vi "Teleop.vi"(10 "Match Info":T7={"Autonomous Elapsed Seconds"=0.0, "TeleOp Elapsed Seconds"=0.0, "Disabled Elapsed Seconds"=0.0, "Visited Autonomous"=FALSE, "Visited TeleOp"=FALSE, "Visited Disabled"=FALSE, "Autonomous Settings"={"Autonomous Style"=enum."Independent", "VI Refnum"=refnum}}, 11 "Call Context":T8) -> ()   [LabVIEW 2015]
doc: "This VI is called for each TeleOp packet received from the DS where the robot is not disabled. It is often used to read from the joysticks and update I/O or to update setpoints for timed control loops. It should complete and return within 20 milliseconds or it may miss DS packets."
uses:
  <vilib>/Rock Robotics/WPI/DriverStation/WPI_DriverStationDerivedRobotMode.ctl
  <vilib>/Rock Robotics/WPI/DriverStation/WPI_DriverStationMatch Info.ctl
  <vilib>/Rock Robotics/Network Tables/NT Read Boolean.vi
  <vilib>/Rock Robotics/Network Tables/NT Read Number.vi
  <vilib>/Rock Robotics/WPI/Utilities/WPI_GetSetVariantRefNum.vi
  <vilib>/Rock Robotics/Network Tables/NT Write Boolean Array.vi
  <vilib>/Rock Robotics/Network Tables/NT Write Numeric Array.vi
  <vilib>/functionblocks/Counter/Timer On Delay/Timer On Delay.vi
  <vilib>/functionblocks/Counter/Pulse Timer/Pulse Timer.vi
  Robot Global Data.vi
  Global 1.vi
  Global 2.vi
  <vilib>/Rock Robotics/Network Tables/NT Write Boolean.vi
  <vilib>/functionblocks/FB Core/FB Core.xnode
  <vilib>/functionblocks/NI_FunctionBlock Libraries.lvlib
panel:
  out "Catapult":T1
  out "DriveTrain Analog":T2
  out "Camera and Joystick Flip Control":T3
  out "Joystick 0 Buttons":T4
  out "Joystick 1 Buttons":T5
  out "Pneumatic Block #1":T6
  out "Arm Angle Ref":dbl
  out "Arm Difference (PID Input)":dbl
  out "Arm Angle":dbl
  out "Sample Slider 0":dbl(slide) scale=0.0..5.0
  out "Sample Boolean 1":bool
  out "Sample Boolean 0":bool
  # "Fwd/Rev"
  # "Left Right"
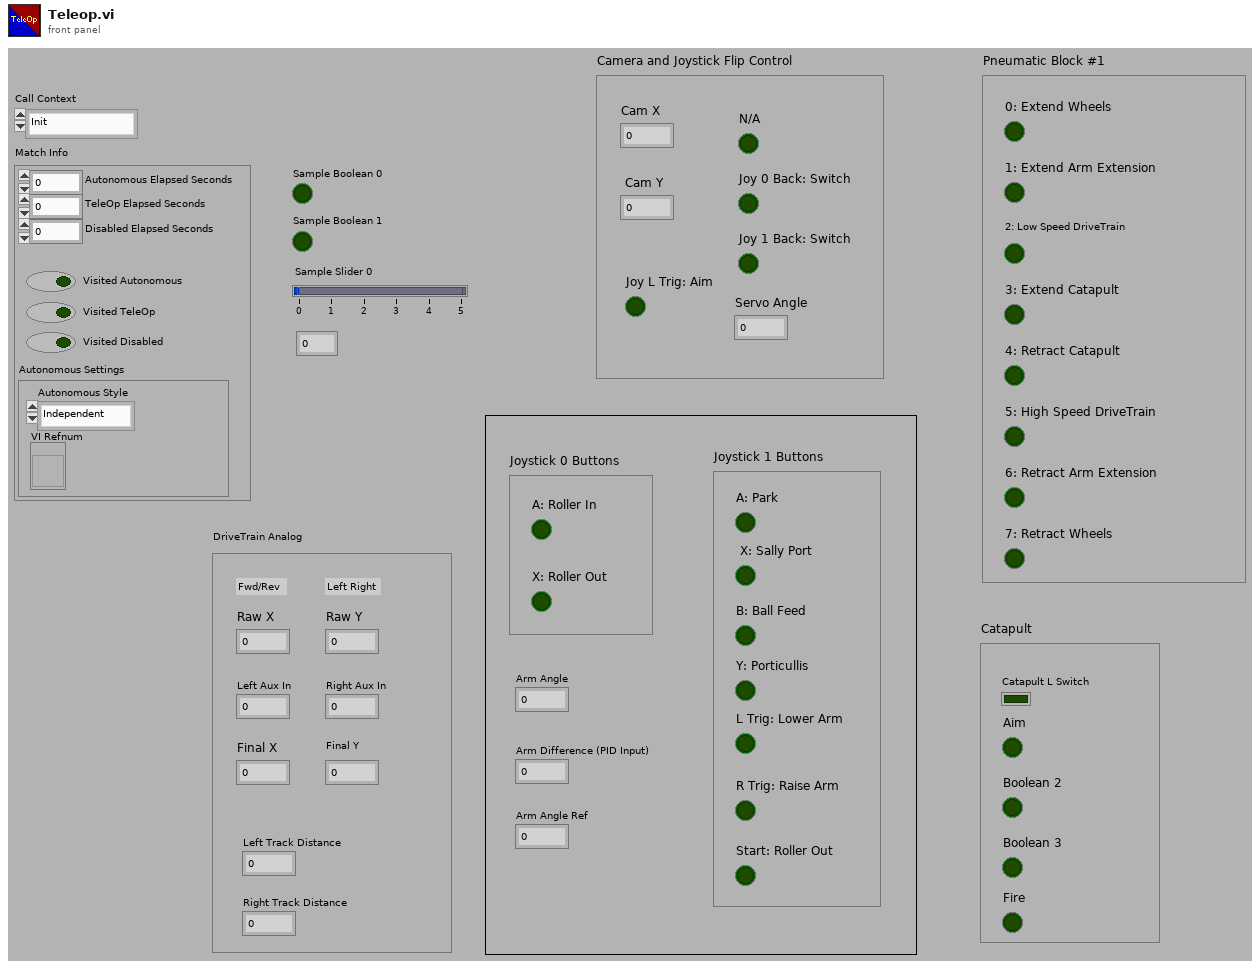
[diagram p1: front panel]
types:
  T1 = cluster{"Catapult L Switch":bool, "Aim":bool, "Boolean 2":bool, "Boolean 3":bool, "Fire":bool}
  T2 = cluster{"Raw X":dbl, "Raw Y":dbl, "Final X":dbl, "Final Y":dbl, "Left Aux In":dbl, "Right Aux In":dbl, "Left Track Distance":dbl, "Right Track Distance":dbl}
  T3 = cluster{"Cam X":dbl, " Cam Y":dbl, "Joy L Trig: Aim":bool, "N/A":bool, "Joy 0 Back: Switch":bool, "Joy 1 Back: Switch":bool, "Servo Angle":dbl}
  T4 = cluster{"A: Roller In":bool, "X: Roller Out":bool}
  T5 = cluster{"A: Park":bool, " X: Sally Port":bool, "B: Ball Feed":bool, "Y: Porticullis":bool, "L Trig: Lower Arm":bool, "R Trig: Raise Arm":bool, "Start: Roller Out":bool}
  T6 = cluster{"0: Extend Wheels ":bool, "1: Extend Arm Extension":bool, "2: Low Speed DriveTrain":bool, "3: Extend Catapult":bool, "4: Retract Catapult":bool, "5: High Speed DriveTrain":bool, "6: Retract Arm Extension":bool, "7: Retract Wheels":bool}
  T7 = typedef "WPI_DriverStationMatch Info.ctl" = cluster{"Autonomous Elapsed Seconds":dbl, "TeleOp Elapsed Seconds":dbl, "Disabled Elapsed Seconds":dbl, "Visited Autonomous":bool, "Visited TeleOp":bool, "Visited Disabled":bool, "Autonomous Settings":cluster{"Autonomous Style":enum16{"Iterative", "Independent"}, "VI Refnum":refnum<vi>}}
  T8 = typedef "WPI_DriverStationDerivedRobotMode.ctl" = enum16{"Init", "Execute", "Stop"}
  T9 = typedef "WPI_JoystickDevRef.ctl" = cluster{"Device":T10}
  T10 = typedef "WPI_JoystickDeviceEnum.ctl" = enum16{"USB 0", "USB 1", "USB 2", "USB 3", "USB 4", "USB 5"}
  T11 = typedef "WPI_EncoderDevRef.ctl" = cluster{"DevStatus":errorcluster, "EncoderIndex":T12, "CounterIndex":T13, "DistancePerCount":dbl, "Decoding Type":T14}
  T12 = typedef "FPGA_EncoderIdx.ctl" = enum8{"Enc 0", "Enc 1", "Enc 2", "Enc 3", "Enc 4", "Enc 5", "Enc 6", "Enc 7", "Invalid"}
  T13 = typedef "FPGA_CounterCtrSystemIndex.ctl" = enum8{"Ctr 0", "Ctr 1", "Ctr 2", "Ctr 3", "Ctr 4", "Ctr 5", "Ctr 6", "Ctr 7", "Invalid"}
  T14 = typedef "WPI_EncoderType.ctl" = enum16{"1x", "2x", "4x"}
  T15 = typedef "WPI_PotentiometerDevRef.ctl" = cluster{"DevStatus":errorcluster, "Analog Channel":T16, "Invert Output":bool}
  T16 = typedef "FPGA_AIChannel.ctl" = enum8{"AI 0", "AI 1", "AI 2", "AI 3", "AI MXP 0", "AI MXP 1", "AI MXP 2", "AI MXP 3", "Invalid"}
  T17 = typedef "WPI_ServoDeviceRef.ctl" = cluster{"DeviceStatus":errorcluster, "PWM Channel":T18, "DeadBand":T19}
  T18 = typedef "FPGA_DIOPWMChannel.ctl" = enum8{"PWM 0", "PWM 1", "PWM 2", "PWM 3", "PWM 4", "PWM 5", "PWM 6", "PWM 7", "PWM 8", "PWM 9", "PWM MXP 0", "PWM MXP 1", "PWM MXP 2", "PWM MXP 3", "PWM MXP 4", "PWM MXP 5", "PWM MXP 6", "PWM MXP 7", "PWM MXP 8", "PWM MXP 9", "Invalid"}
  T19 = typedef "WPI_PWMDeadband.ctl" = cluster{"Name":string, "maxPositivePwm":i32, "minPositivePwm":i32, "centerPwm":i32, "maxNegativePwm":i32, "minNegativePwm":i32, "angularRange":u16}
  T20 = cluster{bool, bool, bool, bool, bool, bool, bool, dbl}
  T21 = cluster{"Cam X Pos":dbl, "Cam Y Pos":dbl, bool, bool, bool, bool, "Value":dbl}
  T22 = cluster{"P":dbl, "I (sec)":dbl, "D (sec)":dbl, dbl}
  T23 = cluster{"Arm Down Speed":dbl, "Arm Up Speed":dbl}
  T24 = typedef "WPI_RelayDevRef.ctl" = cluster{"DevStatus":errorcluster, "Relay Channel":T25, "Relay Direction":T26}
  T25 = typedef "FPGA_DIORelayChannel.ctl" = enum8{"Relay 0", "Relay 1", "Relay 2", "Relay 3", "Invalid"}
  T26 = typedef "WPI_RelayDirection.ctl" = enum16{"Both directions", "Forward only", "Reverse only"}
  T27 = cluster{"Arm Angle":dbl, "Angle Difference (PID Ref)":dbl}
  T28 = cluster{bool, bool, bool, bool, bool, bool, bool}
  T29 = typedef "WPI_RobotDriveDevRef.ctl" = cluster{"DevStatus":errorcluster, "Motors[]":T30[], "Square Inputs":bool, "Max Output":dbl}
  T30 = typedef "WPI_MotorControlDeviceRef.ctl" = cluster{"DeviceStatus":errorcluster, "Type":T31, "PWM":cluster{"PWM Channel":T18, "DeadBand":T19}, "CAN":cluster{"Device Number":u8, "Control Mode":T32, "Semaphore":T33, "Max Vout":dbl, "TalonSRX Control Mode":T34}, "Invert":bool}
  T31 = typedef "WPI_MotorControlType.ctl" = enum16{"PWM", "CAN", "CANTalonSRX"}
  T32 = typedef "WPI_CANJaguar_ControlMode.ctl" = enum8{"Percent VBus", "Current", "Speed", "Position", "Voltage"}
  T33 = typedef "Semaphore RefNum" = refnum<k1>
  T34 = typedef "WPI_CANTalonSRX_APIControlMode.ctl" = enum8{"Percent VBus", "Speed", "Position", "Slave", "Unchanged / Invalid", "Voltage Compensation", "Current", "Motion Profile"}
  T35 = cluster{"Right Joy Out":dbl, "Left Joy Out":dbl, "Fwd/Rev Out":dbl, "Left/Right Out":dbl, "Fwd/Rev Out":dbl, "Left/Right Out":dbl, "Distance":dbl, "Distance":dbl}
  T36 = typedef "WPI_DigitalInputDevRef.ctl" = cluster{"DevStatus":errorcluster, "DIO Channel":T37}
  T37 = typedef "FPGA_DIOChannel.ctl" = enum8{"DIO 0", "DIO 1", "DIO 2", "DIO 3", "DIO 4", "DIO 5", "DIO 6", "DIO 7", "DIO 8", "DIO 9", "DIO MXP 0", "DIO MXP 1", "DIO MXP 2", "DIO MXP 3", "DIO MXP 4", "DIO MXP 5", "DIO MXP 6", "DIO MXP 7", "DIO MXP 8", "DIO MXP 9", "DIO MXP 10", "DIO MXP 11", "DIO MXP 12", "DIO MXP 13", "DIO MXP 14", "DIO MXP 15", "Invalid"}
  T38 = cluster{"Boolean":bool, "Boolean 2":bool, "Boolean 3":bool, "Boolean 4":bool}
  T39 = cluster{string, string, string, string, string, string, string, string}
  T40 = cluster{"Boolean":bool, bool, "Boolean 3":bool, bool, bool, "Boolean 4":bool, bool, "Boolean 2":bool}
  T41 = cluster{"Status 0":bool, "Status 1":bool, "Status 2":bool, "Status 3":bool, "Status 4":bool, "Status 5":bool, "Status 6":bool, "Status 7":bool}
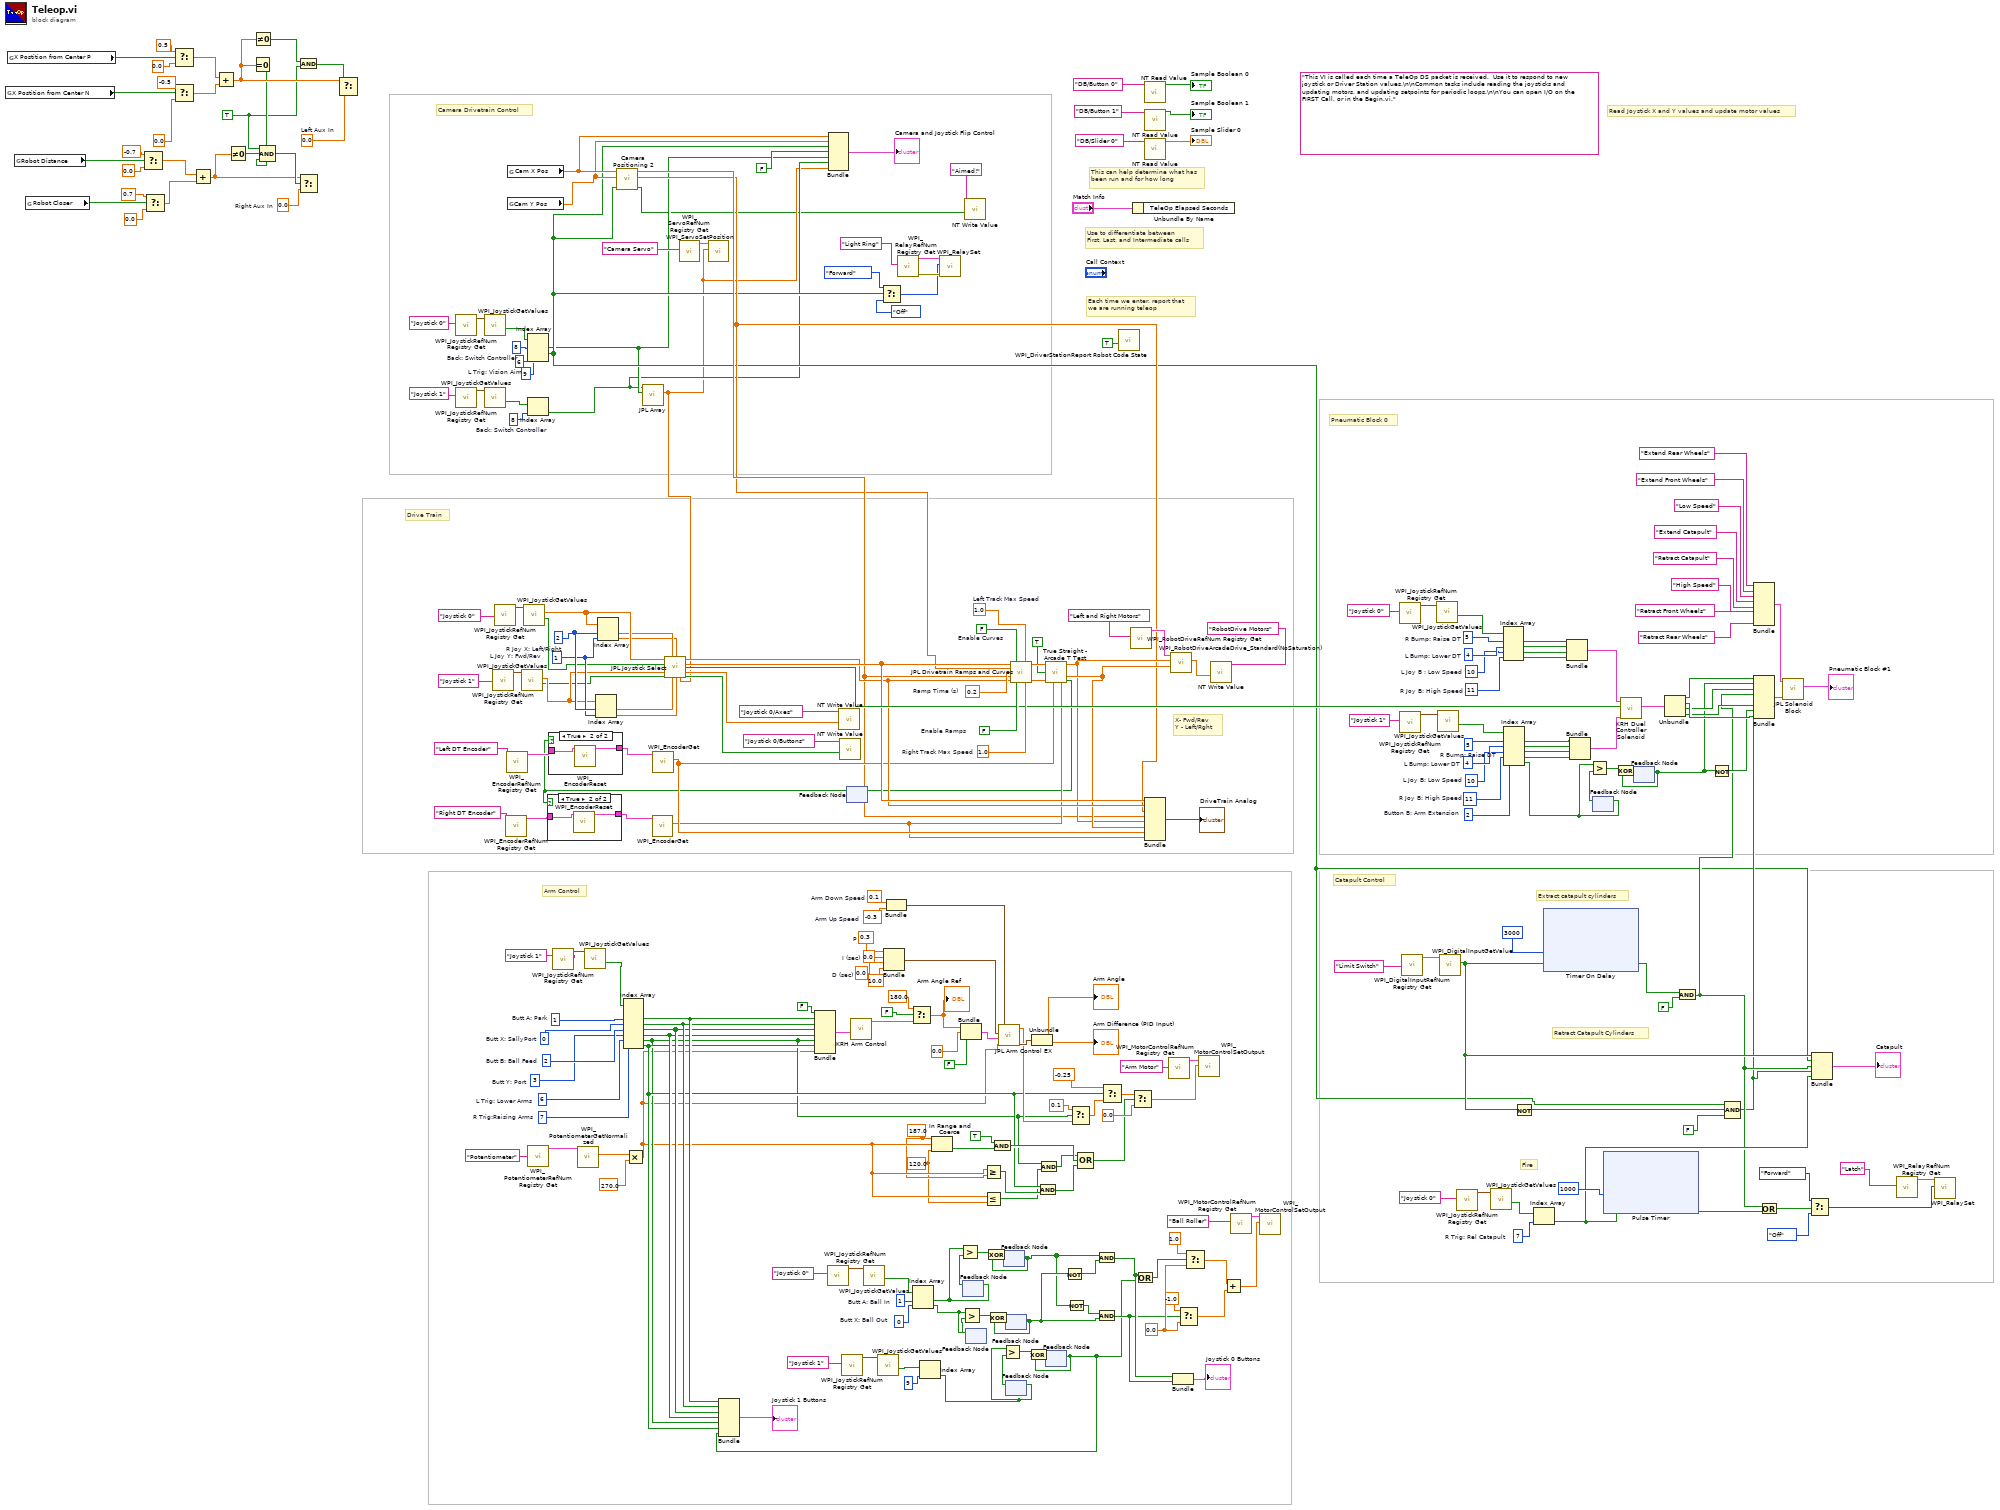
[diagram p0: block diagram]
diagram:
  w33 = TRUE
  w3 = 120.0
  w4 = 187.0
  w91 = 2  # Button B: Arm Extension
  w130 = 0.0
  w104 = 8  # Back: Switch Controller
  w161 = 1  # L Joy Y: Fwd/Rev
  w162 = 2  # R Joy X: Left/Right
  w179 = 11  # R Joy B: High Speed
  w180 = 10  # L Joy B: Low Speed
  w181 = 4  # L Bump: Lower DT
  w182 = 5  # R Bump: Raise DT
  w190 = 8  # Back: Switch Controller
  w105 = 6  # L Trig: Vision Aim
  w210 = 7  # R Trig:Raising Arms
  w211 = 6  # L Trig: Lower Arms
  w138 = 0.0  # Left Aux In
  w137 = 0.0  # Right Aux In
  w214 = 1.0  # Left Track Max Speed
  w216 = 1.0  # Right Track Max Speed
  w215 = FALSE  # Enable Curves
  w218 = 0.2  # Ramp Time (s)
  w217 = FALSE  # Enable Ramps
  w228 = 11  # R Joy B: High Speed
  w229 = 10  # L Joy B : Low Speed
  w231 = 4  # L Bump: Lower DT
  w232 = 5  # R Bump: Raise DT
  w240 = 0.0  # D (sec)
  w239 = 0.0  # I (sec)
  w238 = 0.3  # P
  w242 = -0.3  # Arm Up Speed
  w243 = 0.1  # Arm Down Speed
  w246 = 2  # Butt B: Ball Feed
  w244 = 3  # Butt Y: Port
  w247 = 0  # Butt X: SallyPort
  w248 = 1  # Butt A: Park
  w255 = 0  # Butt X: Ball Out
  w256 = 1  # Butt A: Ball In
  w263 = 7  # R Trig: Rel Catapult
  (unwired) "This VI is called each time a TeleOp DS packet is received.  Use it to respond to new joystick or Driver Station values.\n\nCommon tasks include reading the joysticks and updating motors, and updating setpoints for periodic loops.\n\nYou can open I/O on the FIRST Call, or in the Begin.vi."
  # "Camera Drivetrain Control"
  # "X- Fwd/Rev\nY - Left/Rght"
  # "Retract Catapult Cylinders"
  # "Catapult Control"
  # "Pneumatic Block 0"
  # "Arm Control"
  # "Extract catapult cylinders"
  # "Fire"
  # "Drive Train"
  # "Each time we enter, report that\nwe are running teleop"
  # "Use to differentiate between\nFirst, Last, and Intermediate calls"
  # "This can help determine what has\nbeen run and for how long"
  # "Read Joystick X and Y values and update motor values"
  n1 = global read "Robot Global Data.vi" "X Postition from Center N"() -> (w53:bool)
  n2 = global read "Robot Global Data.vi" "X Postition from Center P"() -> (w54:bool)
  n3 = global read "Robot Global Data.vi" "Robot Distance"() -> (w52:bool)
  n4 = global read "Robot Global Data.vi" "Robot Closer"() -> (w51:bool)
  n5 = Select(t=-0.7, s=w52, f=0.0) -> (s? t:f=w147:dbl)
  n6 = Select(t=0.7, s=w51, f=0.0) -> (s? t:f=w146:dbl)
  n7 = Select(t=0.5, s=w54, f=0.0) -> (s? t:f=w139:dbl)
  n8 = Select(t=-0.5, s=w53, f=0.0) -> (s? t:f=w140:dbl)
  n9 = Add(x=w147, y=w146) -> (x+y=w97:dbl)
  n10 = Add(x=w139, y=w140) -> (x+y=w134:dbl)
  n11 = Not Equal To 0?(x=w97) -> (x != 0?=w135:bool)
  n12 = Equal To 0?(x=w134) -> (x = 0?=w133:bool)
  n13 = Not Equal To 0?(x=w134) -> (x != 0?=w132:bool)
  n14 = Compound Arithmetic op=AND(w33, w135, w133) -> (w136:bool)
  n15 = And(x=w132, y=w33) -> (x .and. y?=w131:bool)
  n16 = Select(t=w97, s=w136, f=w137) -> ()  [unwired: 1 out]
  n17 = Select(t=w134, s=w131, f=w138) -> ()  [unwired: 1 out]
  n18 = call <vilib>:"WPI_JoystickRefNum Registry Get.vi"("refnum name"="Joystick 0") -> ("JoystickDevRef"=w191:T9)  [unwired: 1 in, 9 out]
  n19 = call <vilib>:"WPI_JoystickRefNum Registry Get.vi"("refnum name"="Joystick 1") -> ("JoystickDevRef"=w196:T9)  [unwired: 1 in, 9 out]
  n20 = call <vilib>:"WPI_JoystickGetValues.vi"("JoystickDevRef"=w191) -> ("Buttons"=w189:bool[])  [unwired: 6 in, 4 out]
  n21 = call <vilib>:"WPI_JoystickGetValues.vi"("JoystickDevRef"=w196) -> ("Buttons"=w195:bool[])  [unwired: 6 in, 4 out]
  n22 = call <vilib>:"WPI_JoystickRefNum Registry Get.vi"("refnum name"="Joystick 1") -> ("JoystickDevRef"=w163:T9)  [unwired: 1 in, 9 out]
  n23 = call <vilib>:"WPI_JoystickRefNum Registry Get.vi"("refnum name"="Joystick 0") -> ("JoystickDevRef"=w165:T9)  [unwired: 1 in, 9 out]
  n24 = call <vilib>:"WPI_EncoderRefNum Registry Get.vi"("refnum name"="Right DT Encoder") -> ("EncoderDevRef"=w17:T11)  [unwired: 9 in, 1 out]
  n25 = call <vilib>:"WPI_EncoderRefNum Registry Get.vi"("refnum name"="Left DT Encoder") -> ("EncoderDevRef"=w15:T11)  [unwired: 9 in, 1 out]
  n26 = global read "Global 2.vi" "Cam Y Pos"() -> (w30:dbl)
  n27 = global read "Global 1.vi" "Cam X Pos"() -> (w31:dbl)
  n28 = call <vilib>:"WPI_JoystickGetValues.vi"("JoystickDevRef"=w163) -> ("Buttons"=w155:bool[], "Axes"=w158:dbl[])  [unwired: 6 in, 3 out]
  n29 = call <vilib>:"WPI_JoystickGetValues.vi"("JoystickDevRef"=w165) -> ("Buttons"=w156:bool[], "Axes"=w157:dbl[])  [unwired: 6 in, 3 out]
  n30 = call <vilib>:"WPI_PotentiometerRefNum Registry Get.vi"("refnum name"="Potentiometer") -> ("PotDevRef"=w207:T15)  [unwired: 9 in, 1 out]
  n31 = Index Array(array=w189, index #1=w190, index #2=w105, index #3=9) -> (element #1=w27:bool, element #2=w29:bool)  [unwired: 1 out]
  n32 = Index Array(array=w195, index=w104) -> (element=w26:bool)
  n33 = call <vilib>:"WPI_JoystickRefNum Registry Get.vi"("refnum name"="Joystick 1") -> ("JoystickDevRef"=w249:T9)  [unwired: 1 in, 9 out]
  n34 = call <vilib>:"WPI_PotentiometerGetNormalized.vi"("PotDevRef"=w207) -> ("Normalized Value"=w208:dbl)  [unwired: 8 in, 2 out]
  n35 = call <vilib>:"WPI_JoystickGetValues.vi"("JoystickDevRef"=w249) -> ("Buttons"=w245:bool[])  [unwired: 6 in, 4 out]
  n36 = Index Array(array=w158, index #1=w162, index #2=w161) -> (element #1=w154:dbl, element #2=w153:dbl)
  n37 = Index Array(array=w157, index #1=w162, index #2=w161) -> (element #1=w152:dbl, element #2=w151:dbl)
  n38 = call "Camera Positioning 2.vi"("Aim"=w29, "Y Position"=w30, "X Position"=w31) -> ("Aim Finished"=w23:bool, "Fwd/Rev Out"=w34:dbl, "Left/Right Out"=w35:dbl)  [unwired: 6 in]
  n39 = Index Array(array=w245, index #2=w248, index #3=w247, index #4=w246, index #5=w244, index #6=w211, index #7=w210) -> (element #2=w59:bool, element #3=w58:bool, element #4=w57:bool, element #5=w56:bool, element #6=w6:bool, element #7=w7:bool)  [unwired: 1 in, 1 out]
  n40 = Multiply(x=w208, y=270.0) -> (x*y=w5:dbl)
  n41 = call "JPL Array.vi"("Boolean 2"=w27, "Boolean"=w26) -> ("Value"=w25:dbl)  [unwired: 8 in, 1 out]
  n42 = call "JPL Joystick Select.vi"("Joy 0 Axes"=w157, "Joy 0 Left"=w152, "Joy 0 Right"=w151, "Joy 0 Buttons"=w156, "Joy 1 Axes"=w158, "Joy 1 Buttons"=w155, "Joy 1 Left"=w154, "Joy 1 Right"=w153, "Servo Angle"=w25) -> ("Left Joy Out"=w49:dbl, "Right Joy Out"=w50:dbl, "Joy 0 Selected"=w150:bool, "DS Axes Values"=w160:dbl[], "DS Buttons Values"=w159:bool[])  [unwired: 2 in]
  n43 = call <vilib>:"WPI_ServoRefNum Registry Get.vi"("refnum name"="Camera Servo") -> ("ServoDeviceRef"=w194:T17)  [unwired: 9 in, 1 out]
  n44 = call <vilib>:"WPI_ServoSetPosition.vi"("Position"=w25, "ServoDeviceRef"=w194) -> ()  [unwired: 8 in, 2 out]
  n45 = Bundle(FALSE, w59, w58, w57, w56, w6, w7, w5) -> (w209:T20)  [unwired: 1 in]
  n46 = call <vilib>:"WPI_JoystickRefNum Registry Get.vi"("refnum name"="Joystick 0") -> ("JoystickDevRef"=w258:T9)  [unwired: 1 in, 9 out]
  n47 = Bundle("Cam X Pos"=w31, "Cam Y Pos"=w30, w29, FALSE, w27, w26, "Value"=w25) -> (→"Camera and Joystick Flip Control":T21)  [unwired: 1 in]
  n48 = call-poly <vilib>:"NT Write Value.vi"("Numeric Array"=w160, "Name"="Joystick 0/Axes") -> ()  [unwired: 9 in, 1 out]
  n49 = call-poly <vilib>:"NT Write Value.vi"("Boolean Array"=w159, "Name"="Joystick 0/Buttons") -> ()  [unwired: 9 in, 1 out]
  n50 = call <vilib>:"WPI_JoystickRefNum Registry Get.vi"("refnum name"="Joystick 1") -> ("JoystickDevRef"=w83:T9)  [unwired: 1 in, 9 out]
  n51 = feedback #1() -> (w12:bool)  [unwired: 1 in]
  n52 = case shown="True" w12 {
    tunnel: w17 -> [w280 w282]
    tunnel: [w280 w281] -> w16
    frame False {
    }
    frame True {
      n53 = call <vilib>:"WPI_EncoderReset.vi"("EncoderDevRef"=w282) -> ("EncoderDevRef"=w281:T11)  [unwired: 9 in, 1 out]
    }
  }
  n54 = case shown="True" w12 {
    tunnel: w15 -> [w283 w285]
    tunnel: [w283 w284] -> w14
    frame False {
    }
    frame True {
      n55 = call <vilib>:"WPI_EncoderReset.vi"("EncoderDevRef"=w285) -> ("EncoderDevRef"=w284:T11)  [unwired: 9 in, 1 out]
    }
  }
  n56 = call <vilib>:"WPI_EncoderGet.vi"("EncoderDevRef"=w16) -> ("Distance"=w38:dbl)  [unwired: 5 in, 5 out]
  n57 = call <vilib>:"WPI_EncoderGet.vi"("EncoderDevRef"=w14) -> ("Distance"=w39:dbl)  [unwired: 5 in, 5 out]
  n58 = call "KRH Arm Control.vi"("Button Control"=w209) -> ("Arm Angle"=w68:dbl)  [unwired: 10 in]
  n59 = call <vilib>:"WPI_JoystickGetValues.vi"("JoystickDevRef"=w258) -> ("Buttons"=w257:bool[])  [unwired: 6 in, 4 out]
  n60 = call <vilib>:"WPI_JoystickGetValues.vi"("JoystickDevRef"=w83) -> ("Buttons"=w82:bool[])  [unwired: 6 in, 4 out]
  n61 = Select(t=enum16{"Off", "On", "Forward", "Reverse"}."Forward", s=w29, f=enum16{"Off", "On", "Forward", "Reverse"}."Off") -> (s? t:f=w98:enum16{"Off", "On", "Forward", "Reverse"})
  n62 = Bundle("P"=w238, "I (sec)"=w239, "D (sec)"=w240, 10.0) -> (w20:T22)  [unwired: 1 in]
  n63 = Bundle("Arm Down Speed"=w243, "Arm Up Speed"=w242) -> (w19:T23)  [unwired: 1 in]
  n64 = call <vilib>:"WPI_RelayRefNum Registry Get.vi"("refnum name"="Light Ring") -> ("error out"=w113:errorcluster, "RelayDevRef"=w112:T24)  [unwired: 9 in]
  n65 = Select(t=180.0, s=FALSE, f=w68) -> (s? t:f=w67:dbl)
  "Arm Angle Ref" <- w67
  n66 = Index Array(array=w257, index #1=w256, index #2=w255) -> (element #1=w119:bool, element #2=w116:bool)
  n67 = Index Array(array=w82, index=9) -> (element=w78:bool)
  n68 = In Range and Coerce(upper limit=w4, x=w5, lower limit=w3) -> (In Range?=w75:bool)  [unwired: 1 out]
  n69 = call <vilib>:"WPI_RelaySet.vi"("error in (no error)"=w113, "RelayValue"=w98, "RelayDevRef"=w112) -> ()  [unwired: 7 in, 2 out]
  n70 = Bundle("Arm Angle"=w67, 0.0, FALSE) -> (w21:cluster{"Arm Angle":dbl, dbl, bool})  [unwired: 1 in]
  n71 = feedback-in #2(w119) -> ()
  n72 = feedback #2() -> (w120:bool)  [unwired: 1 in]
  n73 = Greater?(x=w119, y=w120) -> (0:w124:bool)
  n74 = call-poly <vilib>:"NT Write Value.vi"("Boolean"=w23, "Name"="Aimed!") -> ()  [unwired: 9 in, 1 out]
  n75 = feedback-in #3(w116) -> ()
  n76 = feedback #3() -> (w115:bool)  [unwired: 1 in]
  n77 = Greater?(x=w116, y=w115) -> (0:w122:bool)
  n78 = Greater Or Equal?(x=w5, y=w4) -> (x >= y?=w2:bool)
  n79 = Less Or Equal?(x=w5, y=w3) -> (x <= y?=w1:bool)
  n80 = And(x=TRUE, y=w75) -> (x .and. y?=w10:bool)
  n81 = call "JPL Arm Control EX.vi"("Actual Angle"=w5, "Arm Control"=w21, "PID Settings"=w20, "PID Limits"=w19) -> ("Arm Status"=w22:T27, "output"=w18:dbl)  [unwired: 2 in]
  n82 = feedback #4() -> (w117:bool)  [unwired: 1 in]
  n83 = Exclusive Or(1:w117, 2:w124) -> (0:w123:bool)
  n84 = feedback-in #4(w123) -> ()
  n85 = feedback #5() -> (w118:bool)  [unwired: 1 in]
  n86 = Exclusive Or(1:w118, 2:w122) -> (0:w121:bool)
  n87 = feedback-in #5(w121) -> ()
  n88 = feedback #6() -> (w79:bool)  [unwired: 1 in]
  n89 = Greater?(x=w78, y=w79) -> (0:w81:bool)
  n90 = feedback-in #6(w78) -> ()
  n91 = call "JPL Drivetrain Ramps and Curves.vi"("Left Joystick Input"=w50, "Enable Curves"=w215, "Left Max Speed"=w214, "Left Aux In"=w34, "Delay Time (s)"=w218, "Right Aux In"=w35, "Right Joystick Input"=w49, "Enable Ramps"=w217, "Right Max Speed"=w216) -> ("Left Track Out"=w42:dbl, "Right Track Out"=w41:dbl)  [unwired: 5 in]
  n92 = Unbundle(w22) -> ("Arm Angle"=→"Arm Angle":dbl, "Angle Difference (PID Ref)"=→"Arm Difference (PID Input)":dbl)
  n93 = And(x=w7, y=w2) -> (x .and. y?=w8:bool)
  n94 = And(x=w6, y=w1) -> (x .and. y?=w9:bool)
  n95 = call "True Straight - Arcade T Test.vi"("Fwd/Rev Joy"=w42, "Bypass"=TRUE, "Left/Right Joy"=w41, "Left Encoder"=w39, "Right Encoder"=w38) -> ("Fwd/Rev Out"=w36:dbl, "Left/Right Out"=w37:dbl, "Encoder Reset"=w13:bool)  [unwired: 8 in]
  n96 = feedback-in #1(w13) -> ()
  n97 = feedback #7() -> (w55:bool)  [unwired: 1 in]
  n98 = Bundle(w59, w58, w57, w56, w6, w7, w55) -> (→"Joystick 1 Buttons":T28)  [unwired: 1 in]
  n99 = Exclusive Or(1:w55, 2:w81) -> (0:w80:bool)
  n100 = feedback-in #7(w80) -> ()
  n101 = Not(x=w118) -> (.not. x?=w126:bool)
  n102 = Not(x=w117) -> (.not. x?=w125:bool)
  n103 = Select(t=0.1, s=w6, f=w18) -> (s? t:f=w103:dbl)
  n104 = Compound Arithmetic op=OR(w9, w10, w8) -> (w11:bool)
  n105 = And(x=w117, y=w126) -> (x .and. y?=w62:bool)
  n106 = And(x=w125, y=w118) -> (x .and. y?=w61:bool)
  n107 = Select(t=-0.25, s=w7, f=w103) -> (s? t:f=w73:dbl)
  n108 = call <vilib>:"WPI_DriverStationReport Robot Code State.vi"("TeleOp"=TRUE ("Autonomous")) -> ()  [unwired: 10 in, 1 out]
  n109 = call <vilib>:"WPI_RobotDriveRefNum Registry Get.vi"("refnum name"="Left and Right Motors") -> ("RobotDriveDevRef"=w277:T29)  [unwired: 1 in, 9 out]
  n110 = Select(t=w73, s=w11, f=0.0) -> (s? t:f=w72:dbl)
  n111 = Unbundle By Name("Match Info") -> ()  [unwired: 1 out]
  n112 = Or(x=w62, y=w55) -> (x .or. y?=w77:bool)
  n113 = call-poly <vilib>:"NT Read Value.vi"("Name"="DB/Button 0" ("refnum name")) -> ("Boolean"=→"Sample Boolean 0":bool)  [unwired: 9 in, 1 out]
  n114 = call-poly <vilib>:"NT Read Value.vi"("Name"="DB/Slider 0" ("refnum name")) -> ("Numeric"=→"Sample Slider 0":dbl)  [unwired: 9 in, 1 out]
  n115 = call-poly <vilib>:"NT Read Value.vi"("Name"="DB/Button 1" ("refnum name")) -> ("Boolean"=→"Sample Boolean 1":bool)  [unwired: 9 in, 1 out]
  n116 = Bundle("Right Joy Out"=w50, "Left Joy Out"=w49, "Fwd/Rev Out"=w34, "Left/Right Out"=w35, "Fwd/Rev Out"=w36, "Left/Right Out"=w37, "Distance"=w39, "Distance"=w38) -> (→"DriveTrain Analog":T35)  [unwired: 1 in]
  n117 = call <vilib>:"WPI_MotorControlRefNum Registry Get.vi"("refnum name"="Arm Motor") -> ("MotorControlDevRef"=w236:T30)  [unwired: 9 in, 1 out]
  n118 = call <vilib>:"WPI_RobotDriveArcadeDrive_Standard(NoSaturation).vi"("Y axis value"=w37, "X axis value"=w36, "RobotDriveDevRef"=w277) -> ("Motor Values"=w266:dbl[])  [unwired: 1 in, 7 out]
  n119 = Bundle(w62, w61) -> (→"Joystick 0 Buttons":cluster{bool, bool})  [unwired: 1 in]
  n120 = Select(t=-1.0, s=w61, f=w130) -> (s? t:f=w128:dbl)
  n121 = Select(t=1.0, s=w77, f=w130) -> (s? t:f=w129:dbl)
  n122 = call <vilib>:"WPI_MotorControlSetOutput.vi"("Output"=w72, "MotorControlDevRef"=w236) -> ()  [unwired: 7 in, 3 out]
  n123 = call-poly <vilib>:"NT Write Value.vi"("Numeric Array"=w266, "Name"="RobotDrive Motors") -> ()  [unwired: 9 in, 1 out]
  n124 = Add(x=w129, y=w128) -> (x+y=w127:dbl)
  n125 = call <vilib>:"WPI_MotorControlRefNum Registry Get.vi"("refnum name"="Ball Roller") -> ("MotorControlDevRef"=w260:T30)  [unwired: 9 in, 1 out]
  n126 = call <vilib>:"WPI_MotorControlSetOutput.vi"("Output"=w127, "MotorControlDevRef"=w260) -> ()  [unwired: 7 in, 3 out]
  n127 = call <vilib>:"WPI_JoystickRefNum Registry Get.vi"("refnum name"="Joystick 0") -> ("JoystickDevRef"=w234:T9)  [unwired: 1 in, 9 out]
  n128 = call <vilib>:"WPI_JoystickRefNum Registry Get.vi"("refnum name"="Joystick 1") -> ("JoystickDevRef"=w184:T9)  [unwired: 1 in, 9 out]
  n129 = call <vilib>:"WPI_DigitalInputRefNum Registry Get.vi"("refnum name"="Limit Switch") -> ("DigitalInputDevRef"=w200:T36)  [unwired: 9 in, 1 out]
  n130 = call <vilib>:"WPI_JoystickGetValues.vi"("JoystickDevRef"=w234) -> ("Buttons"=w233:bool[])  [unwired: 6 in, 4 out]
  n131 = call <vilib>:"WPI_JoystickGetValues.vi"("JoystickDevRef"=w184) -> ("Buttons"=w183:bool[])  [unwired: 6 in, 4 out]
  n132 = call <vilib>:"WPI_DigitalInputGetValue.vi"("DigitalInputDevRef"=w200) -> ("Value"=w46:bool)  [unwired: 8 in, 2 out]
  n133 = call <vilib>:"WPI_JoystickRefNum Registry Get.vi"("refnum name"="Joystick 0") -> ("JoystickDevRef"=w264:T9)  [unwired: 1 in, 9 out]
  n134 = call <vilib>:"WPI_JoystickGetValues.vi"("JoystickDevRef"=w264) -> ("Buttons"=w204:bool[])  [unwired: 6 in, 4 out]
  n135 = Index Array(array=w233, index #1=w232, index #2=w231, index #3=w229, index #4=w228) -> (element #1=w178:bool, element #2=w177:bool, element #3=w176:bool, element #4=w175:bool)
  n136 = Index Array(array=w183, index #1=w182, index #2=w181, index #3=w180, index #4=w179, index #5=w91) -> (element #1=w174:bool, element #2=w173:bool, element #3=w172:bool, element #4=w171:bool, element #5=w87:bool)
  n137 = Not(x=w46) -> (.not. x?=w70:bool)
  n138 = Index Array(array=w204, index=w263) -> (element=w45:bool)
  n139 = xnode "Timer On Delay"("preset time (ms)"=3000, "input"=w46) -> ("output"=w202:bool)  [unwired: 1 in, 2 out]
  n140 = Bundle(w178, w177, w176, w175) -> (w188:cluster{bool, bool, bool, bool})  [unwired: 1 in]
  n141 = Bundle(w174, w173, w172, w171) -> (w187:cluster{bool, bool, bool, bool})  [unwired: 1 in]
  n142 = feedback #8() -> (w88:bool)  [unwired: 1 in]
  n143 = Greater?(x=w87, y=w88) -> (0:w90:bool)
  n144 = feedback-in #8(w87) -> ()
  n145 = xnode "Pulse Timer"("preset time (ms)"=1000, "input"=w45) -> ("output"=w101:bool)  [unwired: 1 in, 2 out]
  n146 = call "KRH Duel Controller Solenoid.vi"("Joystick 1 Input"=w187, "Joystick Select"=w150, "Joystick 0 Input"=w188) -> ("Solenoid Output"=w186:T38)  [unwired: 8 in]
  n147 = feedback #9() -> (w85:bool)  [unwired: 1 in]
  n148 = Exclusive Or(1:w85, 2:w90) -> (0:w89:bool)
  n149 = feedback-in #9(w89) -> ()
  n150 = Unbundle(w186) -> ("Boolean"=w170:bool, "Boolean 2"=w169:bool, "Boolean 3"=w168:bool, "Boolean 4"=w167:bool)
  n151 = And(x=w202, y=FALSE) -> (x .and. y?=w44:bool)
  n152 = Not(x=w85) -> (.not. x?=w86:bool)
  n153 = Compound Arithmetic op=AND(w29, w70, FALSE) -> (w43:bool)
  n154 = Bundle("Extend Rear Wheels", "Extend Front Wheels", "Low Speed", "Extend Catapult", "Retract Catapult", "High Speed", "Retract Front Wheels", "Retract Rear Wheels") -> (w230:T39)  [unwired: 1 in]
  n155 = Bundle("Boolean"=w170, w85, "Boolean 3"=w168, w44, w43, "Boolean 4"=w167, w86, "Boolean 2"=w169) -> (w71:T40)  [unwired: 1 in]
  n156 = Or(x=w44, y=w101) -> (x .or. y?=w69:bool)
  n157 = call "JPL Solenoid Block.vi"("Boolean Inputs"=w71, "References"=w230) -> ("Status Outputs"=→"Pneumatic Block #1":T41)  [unwired: 9 in]
  n158 = Select(t=enum16{"Off", "On", "Forward", "Reverse"}."Forward", s=w69, f=enum16{"Off", "On", "Forward", "Reverse"}."Off") -> (s? t:f=w108:enum16{"Off", "On", "Forward", "Reverse"})
  n159 = Bundle("Value"=w46, w29, w44, w43, w45) -> (→"Catapult":cluster{"Value":bool, bool, bool, bool, bool})  [unwired: 1 in]
  n160 = call <vilib>:"WPI_RelayRefNum Registry Get.vi"("refnum name"="Latch") -> ("RelayDevRef"=w110:T24)  [unwired: 9 in, 1 out]
  n161 = call <vilib>:"WPI_RelaySet.vi"("RelayValue"=w108, "RelayDevRef"=w110) -> ()  [unwired: 8 in, 2 out]
